vi "Build Server Structure.vi"(8 "error in (no error)":errorcluster, 9 "Folders":T1[](array[typedef]), 10 "Tag Array In":refnum<class "Synchronised Tag.lvclass">[](array[class]), 11 "OPC UA server refnum in":refnum<k21>) -> (0 "error out":errorcluster, 1 "URLs":string[](array[string]), 2 "Tag Array Out":refnum<class "Synchronised Tag.lvclass">[](array[class]), 3 "OPC UA server refnum out":refnum<k21>)   [LabVIEW 2016]
doc: "Creates the item structures in the OPC UA Server"
uses:
  Controls/Folders to Add.ctl
  Sync Tag Class/Synchronised Tag.lvclass
  <vilib>/OPCUA/NI OPC UA Server.lvlib
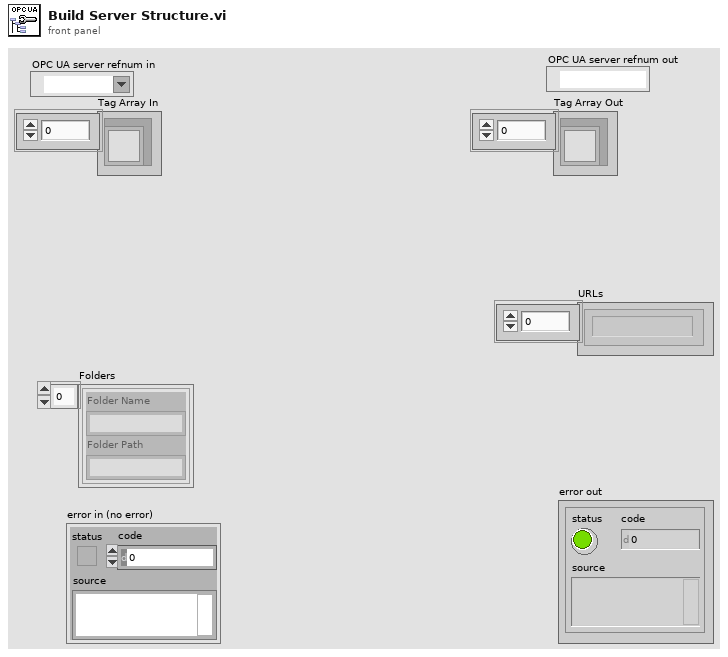
[diagram p1: front panel]
types:
  T1 = typedef "Folders to Add.ctl" = cluster{"Folder Name":string, "Folder Path":string}
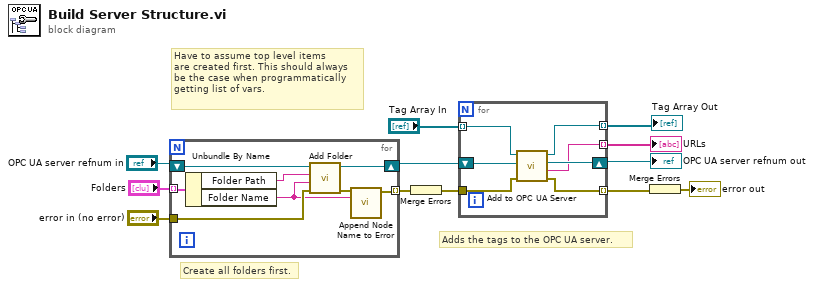
[diagram p0: block diagram]
diagram:
  # "Adds the tags to the OPC UA server."
  # "Create all folders first."
  # "Have to assume top level items\nare created first. This should always\nbe the case when programmatically\ngetting list of vars."
  n1 = for {
    tunnel: "Folders" -> [w15] mode=indexing
    tunnel: "error in (no error)" -> [w19]
    tunnel: [w16] -> w10 mode=indexing
    shift-right: [w18] -> w8
    shift-left: "OPC UA server refnum in" -> [w20]
    n2 = Unbundle By Name(w15) -> ("Folder Path"=w13:string, "Folder Name"=w14:string)
    n3 = call <vilib>:"Add Folder.vi"("error in (no error)"=w19, "folder name"=w14, "parent folder path"=w13, "OPC UA server refnum in"=w20) -> ("error out"=w17:errorcluster, "OPC UA server refnum out"=w18:refnum<k21>)  [unwired: 4 in, 1 out]
    n4 = call "Append Node Name to Error.vi"("Node Name"=w14, "error in (no error)"=w17) -> ("error out"=w16:errorcluster)  [unwired: 9 in]
  }
  n5 = Merge Errors(w10) -> (w9:errorcluster)
  n6 = for {
    tunnel: w9 -> [w27]
    tunnel: [w26] -> w7 mode=indexing
    tunnel: [w22] -> w4 mode=indexing
    shift-right: [w24] -> w5
    shift-left: w8 -> [w25]
    tunnel: [w23] -> w1 mode=indexing
    tunnel: "Tag Array In" -> [w21] mode=indexing
    n7 = call "Add to OPC UA Server.vi"("Error In"=w27, "OPC UA server refnum in"=w25, "Sync Tag In"=w21) -> ("error out"=w26:errorcluster, "URL"=w22:string, "OPC UA server refnum out"=w24:refnum<k21>, "Sync Tag Out"=w23:refnum<class "Synchronised Tag.lvclass">)  [unwired: 5 in]
  }
  "OPC UA server refnum out" <- w5
  "URLs" <- w4
  "Tag Array Out" <- w1
  n8 = Merge Errors(w7) -> (→"error out":errorcluster)
